vi "Build NI Package.vi"() -> ()   [LabVIEW 2021]
uses:
  <vilib>/Wiresmith Technology/G CLI/CLI Class/CLI.lvclass
panel:
  out "Custom Parameters":string[](array[string])
  out "Working Directory":path
  out "error out":errorcluster
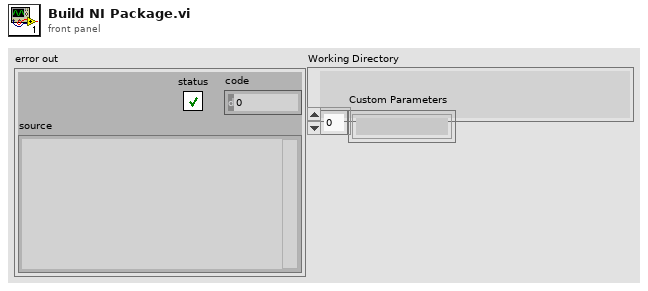
[diagram p1: front panel]
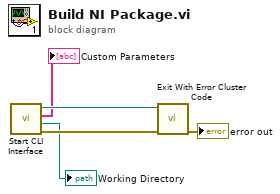
[diagram p0: block diagram]
diagram:
  n1 = call <vilib>:"Start CLI Interface.vi"() -> ("error out"=w4:errorcluster, "Working Directory"=→"Working Directory":path, "Custom Parameters"=→"Custom Parameters":string[], "CLI out"=w5:refnum<class "CLI.lvclass">)  [unwired: 8 in]
  n2 = call <vilib>:"Exit With Error Cluster Code.vi"("error in (no error)"=w4, "CLI in"=w5) -> ("error out"=→"error out":errorcluster)  [unwired: 9 in]
